vi "Initialize.vi"(8 "error in (no error)":errorcluster, 11 "VISA resource name":refnum<visa-resource-name>) -> (0 "error out":errorcluster, 3 "VISA resource name out":refnum<visa-resource-name>)   [LabVIEW 2019, in "Revidyne Generator.lvlib"]
doc: "Establishes communication with the instrument and optionally performs an instrument identification query and/or an instrument reset. It also places the instrument in a default state needed for other instrument driver operations. Therefore, call this VI before calling other instrument driver VIs for this instrument. Generally, you need to call the <b>Initialize</b> VI only once at the beginning of an application."
uses:
  Revidyne Generator.lvlib
  3ce175be-c778-4c90-b2bc-b8e00f0fcd5d.vi
  <vilib>/Instr/_visa.llb/VISA Configure Serial Port (Instr).vi
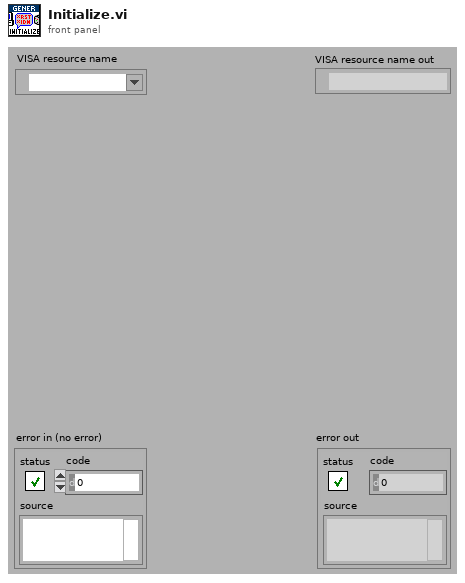
[diagram p1: front panel]
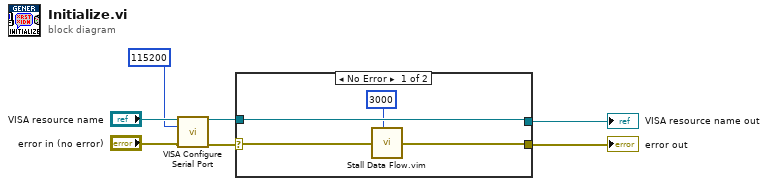
[diagram p0: block diagram]
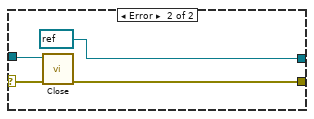
[diagram p2: hidden frame]
diagram:
  n1 = call-poly "VISA Configure Serial Port"("VISA resource name"="VISA resource name", "baud rate (9600)"=u32 115200, "error in (no error)"="error in (no error)") -> ("VISA resource name out"=w5:refnum<visa-resource-name>, "error out"=w2:errorcluster)  [unwired: 11 in]
  n2 = case shown="No Error" w2 {
    selector: w2 -> [w10 w14]
    tunnel: [w11 refnum<visa-resource-name> refnum ("VISA resource name out")] -> w7
    tunnel: [w9 w15] -> w6
    tunnel: w5 -> [w11 w12]
    frame No Error {
      n3 = call "Stall Data Flow.vim"("value in"=w10, "milliseconds to wait"=u32 3000) -> ("value out"=w9:errorcluster)  [unwired: 1 out]
    }
    frame Error {
      n4 = call "Close.vi"("error in (no error)"=w14, "VISA resource name"=w12) -> ("error out"=w15:errorcluster)  [unwired: 9 in]
    }
  }
  "VISA resource name out" <- w7
  "error out" <- w6
